vi "Convert Image pixel.vi"(4 "Channel":string, 6 "image metadata":T2={"serial channel"=0.0, "frame number"=0, "data type"=enum."Frame Start", "width"=0, "height"=0, "image bytes"=0, "total bytes"=0, "little endian"=FALSE, "Status"="Ready for Acquisition"}, 7 "raw display notifier":refnum<notifier>, 8 "error in":errorcluster, 9 "image bytes in":u32, 11 "image pixel data region":refnum<data-value>) -> (0 "error out":errorcluster, 3 "Array":u32[](array[numeric]))   [LabVIEW 2025, in "Automotive Vision.lvclass"]
uses:
  Automotive Vision.lvclass
  Program Files/NI/LVAddons/flexrioii/1/ProjectTemplates/Source/FlexRIO/NI148X/Getting Started/Host/Common/Types/Serial Channel Display Parameters.ctl
  <vilib>/vision/Image Controls.llb/IMAQ Image.ctl
  Program Files/NI/LVAddons/flexrioii/1/ProjectTemplates/Source/FlexRIO/NI148X/Getting Started/Host/Common/Types/RAW Interpretation for Display.ctl
  <instrlib>/FlexRIO/CSI-2/v2/Common/Types/LLP Data Type.ctl
  Automotive Vision.lvclass/Automotive Vision.ctl
  <instrlib>/FlexRIO/Automotive Vision Utility/v1/Host/Automotive Vision Utility.lvlib
  Program Files/NI/LVAddons/flexrioii/1/ProjectTemplates/Source/FlexRIO/NI148X/Getting Started/Host/Common/GettingStarted_Common_148X_Host.lvlib
  <instrlib>/FlexRIO/CSI-2/v2/Common/NI CSI-2 API Common v2.lvlib
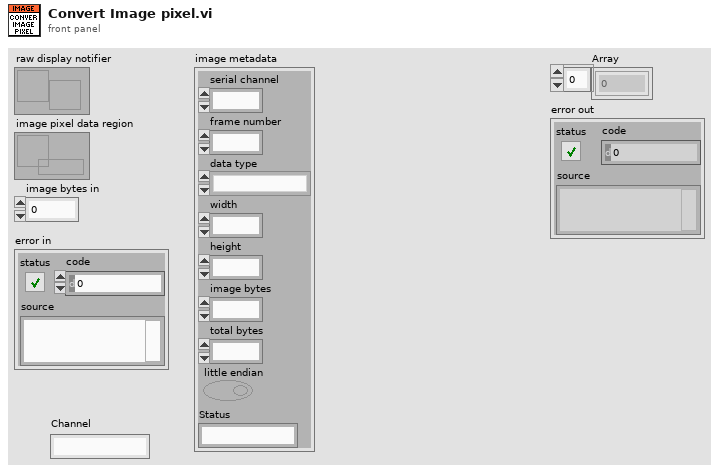
[diagram p1: front panel]
types:
  T1 = typedef "NI CSI-2 API Common v2.lvlib/LLP Data Type.ctl" = enum8{"Frame Start", "Frame End", "Line Start", "Line End", "End of Transmission", "Reserved 0", "Reserved 1", "Reserved 2", "Generic Short Packet 1", "Generic Short Packet 2", "Generic Short Packet 3", "Generic Short Packet 4", "Generic Short Packet 5", "Generic Short Packet 6", "Generic Short Packet 7", "Generic Short Packet 8", "Null", "Blanking Data", "Embedded 8-bit non Image Data", "Generic Long Packet 1", "Generic Long Packet 2", "Generic Long Packet 3", "Generic Long Packet 4", "Reserved 3", "YUV420 8-bit", "YUV420 10-bit", "Legacy YUV420 8-bit", "Reserved 4", "YUV420 8-bit Chroma Shifted", "YUV420 10-bit Chroma Shifted", "YUV422 8-bit", "YUV422 10-bit", "RGB444", "RGB555", "RGB565", "RGB666", "RGB888", "Reserved 5", "Reserved 6", "RAW 24", "RAW 6", "RAW 7", "RAW 8", "RAW 10", "RAW 12", "RAW 14", "RAW 16", "RAW 20", "User Defined 8-bit Data 1", "User Defined 8-bit Data 2", "User Defined 8-bit Data 3", "User Defined 8-bit Data 4", "User Defined 8-bit Data 5", "User Defined 8-bit Data 6", "User Defined 8-bit Data 7", "User Defined 8-bit Data 8", "USL Command", "Reserved 7", "Reserved 8", "Reserved 9", "Reserved 10", "Reserved 11", "Reserved 12", "LRTE EPD Spacer"}
  T2 = cluster{"serial channel":fxp<+,3,3>, "frame number":u16, "data type":T1, "width":u16, "height":u16, "image bytes":u32, "total bytes":u32, "little endian":bool, "Status":string}
  T3 = typedef "GettingStarted_Common_148X_Host.lvlib/Serial Channel Display Parameters.ctl" = cluster{"images":cluster{"grayscale":T4, "color":T4}, "RAW parameters":cluster{"interpretation":T5, "bayer parameters":cluster{"pattern":i32, "algorithm":i32, "red gain":dbl, "green gain":dbl, "blue gain":dbl}}}
  T4 = typedef "IMAQ Image.ctl" = refnum<image>
  T5 = typedef "GettingStarted_Common_148X_Host.lvlib/RAW Interpretation for Display.ctl" = enum16{"Grayscale", "Bayer", "RGB", "YUV422", "YUV420", "Legacy YUV420"}
  T6 = enum8{"Frame Start", "Frame End", "Line Start", "Line End", "End of Transmission", "Reserved 0", "Reserved 1", "Reserved 2", "Generic Short Packet 1", "Generic Short Packet 2", "Generic Short Packet 3", "Generic Short Packet 4", "Generic Short Packet 5", "Generic Short Packet 6", "Generic Short Packet 7", "Generic Short Packet 8", "Null", "Blanking Data", "Embedded 8-bit non Image Data", "Generic Long Packet 1", "Generic Long Packet 2", "Generic Long Packet 3", "Generic Long Packet 4", "Reserved 3", "YUV420 8-bit", "YUV420 10-bit", "Legacy YUV420 8-bit", "Reserved 4", "YUV420 8-bit Chroma Shifted", "YUV420 10-bit Chroma Shifted", "YUV422 8-bit", "YUV422 10-bit", "RGB444", "RGB555", "RGB565", "RGB666", "RGB888", "Reserved 5", "Reserved 6", "RAW 24", "RAW 6", "RAW 7", "RAW 8", "RAW 10", "RAW 12", "RAW 14", "RAW 16", "RAW 20", "User Defined 8-bit Data 1", "User Defined 8-bit Data 2", "User Defined 8-bit Data 3", "User Defined 8-bit Data 4", "User Defined 8-bit Data 5", "User Defined 8-bit Data 6", "User Defined 8-bit Data 7", "User Defined 8-bit Data 8", "USL Command", "Reserved 7", "Reserved 8", "Reserved 9", "Reserved 10", "Reserved 11", "Reserved 12", "LRTE EPD Spacer"}
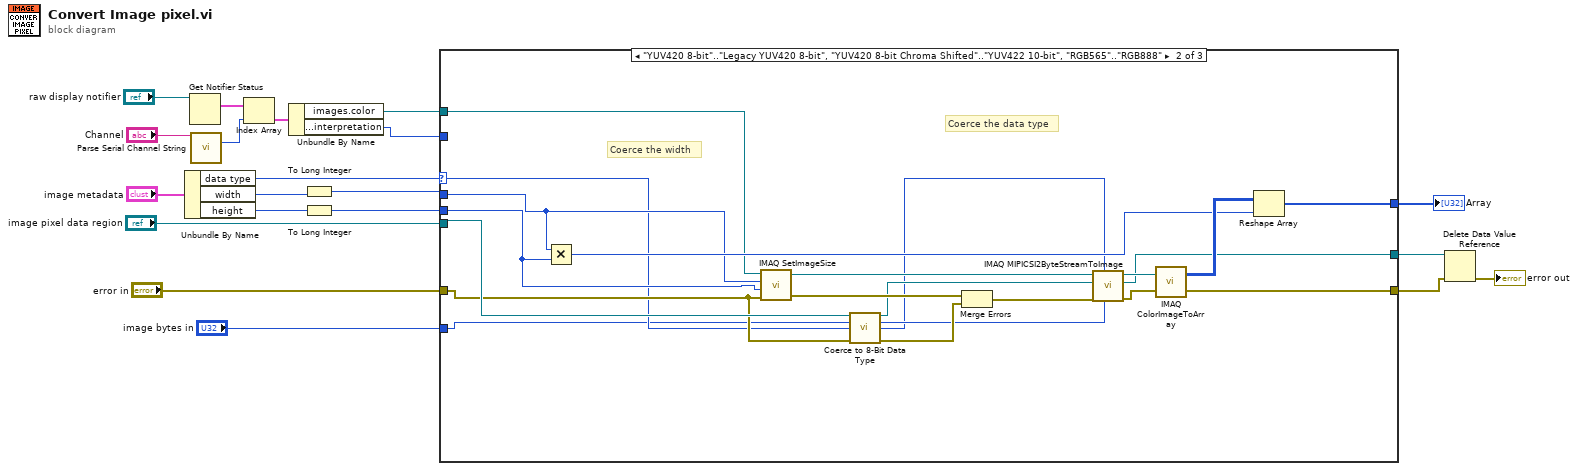
[diagram p0: block diagram]
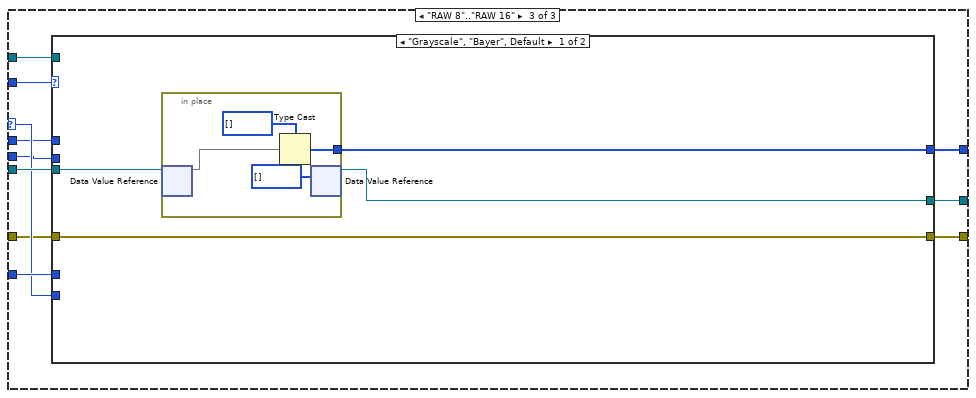
[diagram p3: hidden frame]
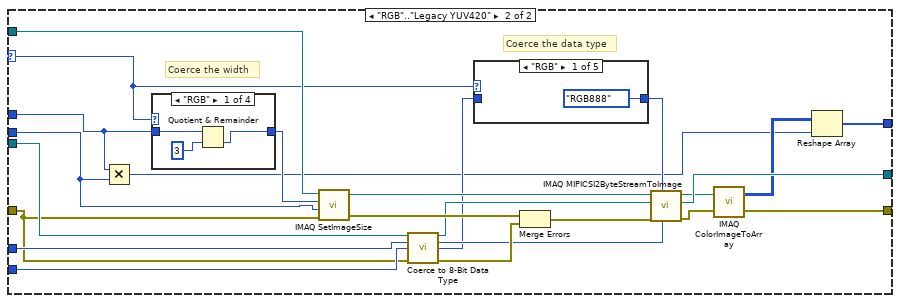
[diagram p4: hidden frame]
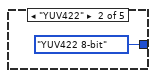
[diagram p5: hidden frame]
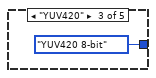
[diagram p6: hidden frame]
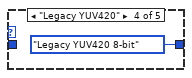
[diagram p7: hidden frame]
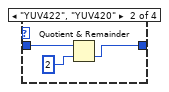
[diagram p9: hidden frame]
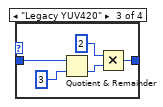
[diagram p10: hidden frame]
diagram:
  n1 = Unbundle By Name("image metadata") -> ("data type"=w19:T1, "width"=w4:u16, "height"=w2:u16)
  n2 = Get Notifier Status(notifier="raw display notifier") -> (current notification=w18:T3[])  [unwired: 1 in, 4 out]
  n3 = call <instrlib>:"Parse Serial Channel String.vi"("serial channel string"="Channel") -> ("channel number"=w6:i32)  [unwired: 13 in, 1 out]
  n4 = Index Array(array=w18, index=w6) -> (element=w16:T3)
  n5 = Unbundle By Name(w16) -> ("images.color"=w11:T4, "RAW parameters.interpretation"=w15:T5)
  n6 = To Long Integer(number=w4) -> (32bit integer=w3:i32)
  n7 = To Long Integer(number=w2) -> (32bit integer=w1:i32)
  n8 = case shown="\"YUV420 8-bit\"..\"Legacy YUV420 8-bit\", \"YUV420 8-bit Chroma Shifted\"..\"YUV422 10-bit\", \"RGB565\"..\"RGB888\"" w19 {
    selector: w19 -> [_ w24 w48]
    tunnel: w15 -> [_ _ w54]
    tunnel: "image pixel data region" -> [w21 w31 w53]
    tunnel: [_ w29 w52] -> w12
    tunnel: [w21 w30 w51] -> w13
    tunnel: w11 -> [_ w33 w50]
    tunnel: "image bytes in" -> [_ w23 w49]
    tunnel: w3 -> [_ w27 w47]
    tunnel: "error in" -> [w22 w25 w46]
    tunnel: w1 -> [_ w32 w45]
    tunnel: [w22 w28 w44] -> w8
    frame "Frame Start", Default {
    }
    frame "YUV420 8-bit".."Legacy YUV420 8-bit", "YUV420 8-bit Chroma Shifted".."YUV422 10-bit", "RGB565".."RGB888" {
      # "Coerce the data type"
      # "Coerce the width"
      n9 = Multiply(x=w27, y=w32) -> (x*y=w34:i32)
      n10 = call "IMAQ SetImageSize"("error in (no error)"=w25, "Y Resolution"=w32, "X Resolution"=w27, "Image"=w33) -> ("error out"=w42:errorcluster, "Image Out"=w43:T4)  [unwired: 1 in]
      n11 = call "Coerce to 8-Bit Data Type.vi"("image pixel data region in"=w31, "image bytes in"=w23, "data type in"=w24, "error in (no error)"=w25) -> ("image pixel data region out"=w38:refnum<data-value>, "image bytes out"=w39:u32, "data type out"=w26:T6, "error out"=w40:errorcluster)  [unwired: 8 in]
      n12 = Merge Errors(w42, w40) -> (w41:errorcluster)
      n13 = call "IMAQ MIPICSI2ByteStreamToImage"("Bytes to Copy"=w39, "Format"=w26, "error in (no error)"=w41, "Byte Stream In"=w38, "Image In"=w43) -> ("error out"=w36:errorcluster, "Byte Stream Out"=w30:refnum<data-value>, "Image Out"=w37:T4)  [unwired: 3 in, 1 out]
      n14 = call "IMAQ ColorImageToArray"("Image"=w37, "error in (no error)"=w36) -> ("Image Pixels (U32)"=w35:u32[][], "error out"=w28:errorcluster)  [unwired: 2 in, 1 out]
      n15 = Reshape Array(w35, w34) -> (w29:u32[])
    }
    frame "RAW 8".."RAW 16" {
      n16 = case shown="\"Grayscale\", \"Bayer\", Default" w54 {
        selector: w54 -> [_ w75]
        tunnel: w53 -> [w58 w74]
        tunnel: [w57 w66] -> w52
        tunnel: [w56 w77] -> w51
        tunnel: w50 -> [_ w76]
        tunnel: w49 -> [_ w73]
        tunnel: w48 -> [_ w72]
        tunnel: w47 -> [_ w65]
        tunnel: w46 -> [w55 w71]
        tunnel: w45 -> [_ w64]
        tunnel: [w55 w67] -> w44
        frame "Grayscale", "Bayer", Default {
          n17 = in-place {
            in-place-border: [w60] -> w57
            n18 = in-place-dvr #1(w58) -> (w62:u8[])  [unwired: 1 out]
            n19 = Type Cast(type=u32[] [], x=w62) -> (*(type *) &x=w60:u32[])
            n20 = in-place-dvr #1(u8[] [] ("data value")) -> (w56:refnum<data-value>)  [unwired: 1 out]
          }
        }
        frame "RGB".."Legacy YUV420" {
          # "Coerce the data type"
          # "Coerce the width"
          n21 = Multiply(x=w65, y=w64) -> (x*y=w63:i32)
          n22 = case shown="\"RGB\"" w75 {
            tunnel: w65 -> [w93 w96 w102 w103]
            tunnel: [w92 w95 w99 w103] -> w80
            frame "RGB" {
              n23 = Quotient & Remainder(x=w93, y=3) -> (floor(x/y)=w92:i32)  [unwired: 1 out]
            }
            frame "YUV422", "YUV420" {
              n24 = Quotient & Remainder(x=w96, y=2) -> (floor(x/y)=w95:i32)  [unwired: 1 out]
            }
            frame "Legacy YUV420" {
              n25 = Quotient & Remainder(x=w102, y=3) -> (floor(x/y)=w100:i32)  [unwired: 1 out]
              n26 = Multiply(x=2, y=w100) -> (x*y=w99:i32)
            }
            frame Default {
            }
          }
          n27 = call "IMAQ SetImageSize"("error in (no error)"=w71, "Y Resolution"=w64, "X Resolution"=w80, "Image"=w76) -> ("error out"=w85:errorcluster, "Image Out"=w86:T4)  [unwired: 1 in]
          n28 = call "Coerce to 8-Bit Data Type.vi"("image pixel data region in"=w74, "image bytes in"=w73, "data type in"=w72, "error in (no error)"=w71) -> ("image pixel data region out"=w81:refnum<data-value>, "image bytes out"=w82:u32, "data type out"=w78:T6, "error out"=w83:errorcluster)  [unwired: 8 in]
          n29 = case shown="\"RGB\"" w75 {
            tunnel: w78 -> [_ _ _ _ w91]
            tunnel: [T6."RGB888" ("data type") T6."YUV422 8-bit" ("data type") T6."YUV420 8-bit" ("data type") T6."Legacy YUV420 8-bit" ("data type") w91] -> w79
            frame "RGB" {
            }
            frame "YUV422" {
            }
            frame "YUV420" {
            }
            frame "Legacy YUV420" {
            }
            frame Default {
            }
          }
          n30 = Merge Errors(w85, w83) -> (w84:errorcluster)
          n31 = call "IMAQ MIPICSI2ByteStreamToImage"("Bytes to Copy"=w82, "Format"=w79, "error in (no error)"=w84, "Byte Stream In"=w81, "Image In"=w86) -> ("error out"=w69:errorcluster, "Byte Stream Out"=w77:refnum<data-value>, "Image Out"=w70:T4)  [unwired: 3 in, 1 out]
          n32 = call "IMAQ ColorImageToArray"("Image"=w70, "error in (no error)"=w69) -> ("Image Pixels (U32)"=w68:u32[][], "error out"=w67:errorcluster)  [unwired: 2 in, 1 out]
          n33 = Reshape Array(w68, w63) -> (w66:u32[])
        }
      }
    }
  }
  "Array" <- w12
  n34 = Delete Data Value Reference(data value reference=w13, error in=w8) -> (error out=→"error out":errorcluster)  [unwired: 1 out]
